vi "Read without Trigger Model (Multiple Points).vi"(6 "Buffer Elements":u16(ring) items=["Date", "Extra", "Formatted", "Fractional", "Relative", "Seconds", "Status", "Time", "Timestamp", "Unit"], 8 "error in (no error)":errorcluster, 9 "Timeout (10000 ms)":i32=10000 format="%#.6g", 10 "Buffer Name":string="defbuffer1", 11 "VISA resource name":refnum<visa-resource-name>) -> (0 "error out":errorcluster, 1 "Element Value":string[](array[string]), 2 "Measurements":dbl[](array[numeric]), 3 "VISA resource name out":refnum<visa-resource-name>)   [LabVIEW 2018, in "Keithley DMM7512.lvlib"]
doc: "This VI makes readings using the active measure function and stores them in the reading buffer. Reads and returns multiple measurements from the instrument specified buffer."
uses:
  <instrlib>/Keithley DMM7512/Keithley DMM7512.lvlib
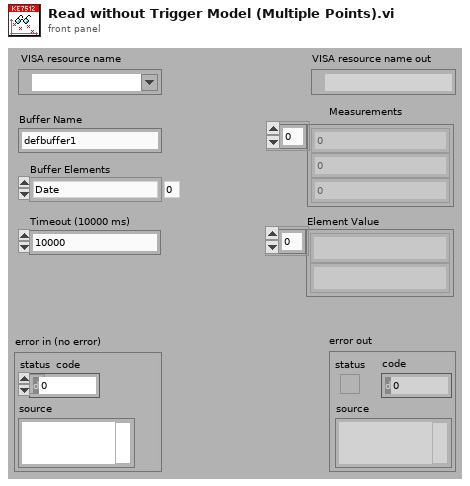
[diagram p1: front panel]
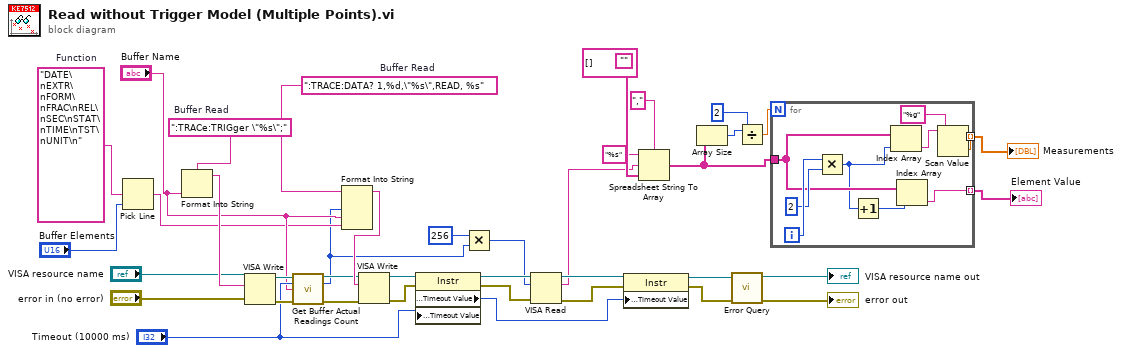
[diagram p0: block diagram]
diagram:
  w10 = ":TRACe:TRIGger \"%s\";"  # Buffer Read
  (unwired) ""
  w25 = "DATE\nEXTR\nFORM\nFRAC\nREL\nSEC\nSTAT\nTIME\nTST\nUNIT\n"  # Function
  w28 = ":TRACE:DATA? 1,%d,\"%s\",READ, %s"  # Buffer Read
  n1 = Pick Line(multi-line string=w25, line index="Buffer Elements") -> (output string=w4:string)  [unwired: 1 out]
  n2 = Format Into String(format string=w10, "Buffer Name") -> (resulting string=w9:string)  [unwired: 2 in, 1 out]
  n3 = VISA Write(VISA resource name="VISA resource name", write buffer=w9, error in (no error)="error in (no error)") -> (VISA resource name out=w12:refnum<visa-resource-name>, error out=w11:errorcluster)  [unwired: 1 out]
  n4 = call <instrlib>:"Get Buffer Actual Readings Count.vi"("VISA resource name"=w12, "Timeout (10000 ms)"="Timeout (10000 ms)", "Buffer Name (defbuffer1)"="Buffer Name", "error in (no error)"=w11) -> ("VISA resource name out"=w13:refnum<visa-resource-name>, "Actual Readings"=w2:i32, "error out"=w14:errorcluster)  [unwired: 9 in]
  n5 = Format Into String(format string=w28, w2, "Buffer Name", w4) -> (resulting string=w27:string)  [unwired: 2 in, 1 out]
  n6 = VISA Write(VISA resource name=w13, write buffer=w27, error in (no error)=w14) -> (VISA resource name out=w37:refnum<visa-resource-name>, error out=w36:errorcluster)  [unwired: 1 out]
  n7 = property class="Instr"(reference=w37, error in=w36, "General Settings:Timeout Value"="Timeout (10000 ms)") -> (reference out=w35:refnum<visa-resource-name>, error out=w34:errorcluster, "General Settings:Timeout Value"=w29:u32)
  n8 = Multiply(x=256, y=w2) -> (x*y=w3:i32)
  n9 = VISA Read(VISA resource name=w35, byte count=w3, error in (no error)=w34) -> (VISA resource name out=w33:refnum<visa-resource-name>, read buffer=w15:string, error out=w31:errorcluster)  [unwired: 1 out]
  n10 = property class="Instr"(reference=w33, error in=w31, "General Settings:Timeout Value"=w29) -> (reference out=w32:refnum<visa-resource-name>, error out=w30:errorcluster)
  n11 = Spreadsheet String To Array(delimiter (Tab)=",", format string="%s", spreadsheet string=w15, array type (2D Dbl)=string[] []) -> (array=w22:string[])
  n12 = Array Size(array=w22) -> (size(s)=w20:i32)
  n13 = call <instrlib>:"Error Query.vi"("error in (no error)"=w30, "VISA resource name"=w32) -> ("error out"=→"error out":errorcluster, "VISA resource name out"=→"VISA resource name out":refnum<visa-resource-name>)  [unwired: 6 in, 2 out]
  n14 = Divide(x=w20, y=2) -> (x/y=w18:dbl)
  n15 = for {
    N: w18 -> [_]
    tunnel: w22 -> [w46]
    tunnel: [w41] -> w17 mode=indexing
    tunnel: [w44] -> w16 mode=indexing
    i -> [w48]
    n16 = Multiply(x=w48, y=2) -> (x*y=w40:i32)
    n17 = Increment(x=w40) -> (x+1=w45:i32)
    n18 = Index Array(array=w46, index=w40) -> (element=w43:string)
    n19 = Index Array(array=w46, index=w45) -> (element=w44:string)
    n20 = Scan Value(string=w43, format string="%g") -> (value=w41:dbl)  [unwired: 1 in, 1 out]
  }
  "Measurements" <- w17
  "Element Value" <- w16
